vi "Initialize ConsoleView.vi"(8 "error in (no error)":errorcluster, 11 "ConsoleView in":refnum<class "ConsoleView.lvclass">) -> (0 "error out":errorcluster, 3 "ConsoleView out":refnum<class "ConsoleView.lvclass">)   [LabVIEW 2019, in "ConsoleView.lvlib" / "ConsoleView.lvclass"]
uses:
  <vilib>/gpm_packages/@cs/event-logger/Source/ConsoleView/View/ConsoleView.lvclass
  <vilib>/gpm_packages/@cs/event-logger/Source/Composed Log/Types/MessageCluster.ctl
  <vilib>/gpm_packages/@cs/event-logger/Source/Composed Log/Types/Log Packet.ctl
  <vilib>/gpm_packages/@cs/event-logger/Source/Composed Log/Types/Log Level.ctl
  <vilib>/gpm_packages/@cs/event-logger/Source/ConsoleView/View/TypeDef/FilterConfig.ctl
  <vilib>/gpm_packages/@cs/event-logger/Source/ConsoleView/View/ConsoleView.lvclass/ConsoleView.ctl
  <vilib>/gpm_packages/@cs/event-logger/Source/Composed Log/Composed Log.lvlib
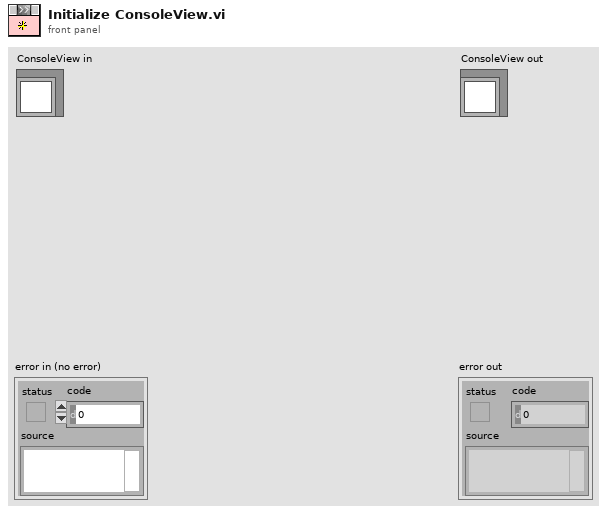
[diagram p1: front panel]
types:
  T1 = typedef "ConsoleView.lvlib/ConsoleView.lvclass/FilterConfig.ctl" = cluster{"Level Filter":cluster{"Warning":bool, "Debug":bool, "Info":bool, "Error":bool, "Critical":bool}, "Source Filter":cluster{"Source":string, "Exclude Match?":bool, "Exact Match?":bool}, "Keyword Filter":cluster{"Keywords":string[], "Exclude Match?":bool}}
  T2 = typedef "Composed Log.lvlib/Log Packet.ctl" = cluster{"Data To Log":string, "Source":string, "Event Level":T3, "Event Time":timestamp}
  T3 = typedef "Composed Log.lvlib/Log Level.ctl" = enum16{"Debug", "Info", "Warning", "Error", "Critical"}
  T4 = typedef "Composed Log.lvlib/MessageCluster.ctl" = cluster{"Message":string, "Data":variant}
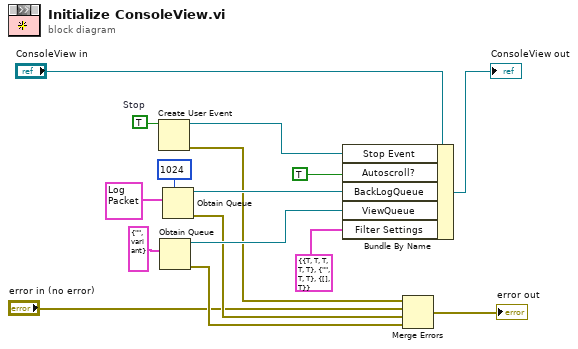
[diagram p0: block diagram]
diagram:
  w4 = TRUE  # Stop
  n1 = Create User Event(user event datatype=w4) -> (user event=w3:refnum<user-event>, error out=w2:errorcluster)  [unwired: 1 in]
  n2 = Obtain Queue(element data type=T4 {"Message"="", "Data"=variant} ("Cluster")) -> (queue out=w10:refnum<queue>, error out=w8:errorcluster)  [unwired: 4 in, 1 out]
  n3 = Obtain Queue(max queue size (-1, unlimited)=1024, element data type=T2 {"Data To Log"="", "Source"="", "Event Level"=enum."Debug", "Event Time"=timestamp(0 s since 1904-01-01)} ("Log Packet")) -> (queue out=w11:refnum<queue>, error out=w9:errorcluster)  [unwired: 3 in, 1 out]
  n4 = Bundle By Name(cluster="ConsoleView in", "Stop Event"=w3, "Autoscroll?"=TRUE, "BackLogQueue"=w11, "ViewQueue"=w10, "Filter Settings"=T1 {"Level Filter"={"Warning"=TRUE, "Debug"=TRUE, "Info"=TRUE, "Error"=TRUE, "Critical"=TRUE}, "Source Filter"={"Source"="", "Exclude Match?"=TRUE, "Exact Match?"=TRUE}, "Keyword Filter"={"Keywords"=[], "Exclude Match?"=TRUE}}) -> (→"ConsoleView out":refnum<class "ConsoleView.lvclass">)
  n5 = Merge Errors(w2, "error in (no error)", w9, w8) -> (→"error out":errorcluster)
